vi "CFG_write.vi"(8 "error in":errorcluster, 10 "default folder":path, 11 "config file":path) -> (0 "error out":errorcluster, 3 "config file dup":path)   [LabVIEW 2015]
uses:
  <vilib>/Utility/config.llb/Write Key (Path).vi
  <vilib>/Utility/config.llb/NI_LVConfig.lvlib
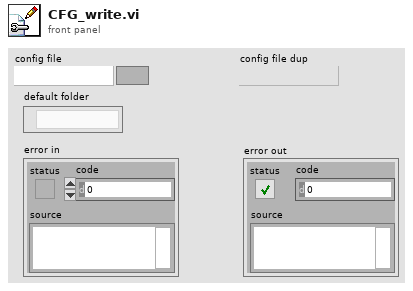
[diagram p1: front panel]
types:
  T1 = typedef "NI_LVConfig.lvlib/Config Data RefNum.ctl" = refnum<k1>
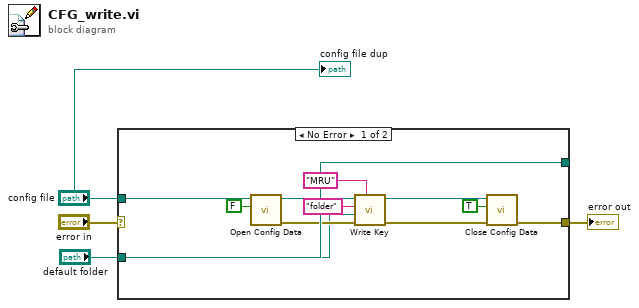
[diagram p0: block diagram]
diagram:
  n1 = case shown="No Error" "error in" {
    tunnel: [w15 _] -> w4
    tunnel: "default folder" -> [_ _]
    tunnel: "config file" -> [w7 _]
    tunnel: "default folder" -> [w6 _]
    frame No Error {
      n2 = call <vilib>:"Open Config Data.vi"("create file if necessary (T)"=FALSE, "configuration file path"=w7) -> ("error out"=w10:errorcluster, "refnum"=w8:T1)  [unwired: 7 in, 1 out]
      n3 = call-poly <vilib>:"Write Key.vi"("section"="MRU", "error in (no error)"=w10, "value"=w6, "key"="folder", "refnum"=w8) -> ("error out"=w11:errorcluster, "refnum out"=w9:T1)  [unwired: 4 in, 1 out]
      n4 = call <vilib>:"Close Config Data.vi"("error in (no error)"=w11, "write file if changed (T)"=TRUE, "refnum"=w9) -> ("error out"=w15:errorcluster)  [unwired: 7 in, 1 out]
    }
    frame Error {
    }
  }
  "error out" <- w4
  "config file dup" <- "config file"
